vi "Autonomous Independent.vi"() -> ()   [LabVIEW 2019]
doc: "This VI is called when autonomous begins, and will automatically be terminated when autonomous ends. You can carry out timed or sensor driven robot movement independently without needing to return to the caller."
uses:
  <vilib>/Rock Robotics/WPI/Utilities/WPI_GetSetVariantRefNum.vi
  <vilib>/Rock Robotics/Network Tables/NT Write Numeric Array.vi
  <vilib>/Rock Robotics/Network Tables/NT Read String.vi
panel:
  out "Ultrasonic 2":dbl
  out "Ultrasonic":dbl
  out "Degrees 2":dbl(knob) scale=0.0..360.0
  out "Degrees":dbl(knob) scale=0.0..360.0
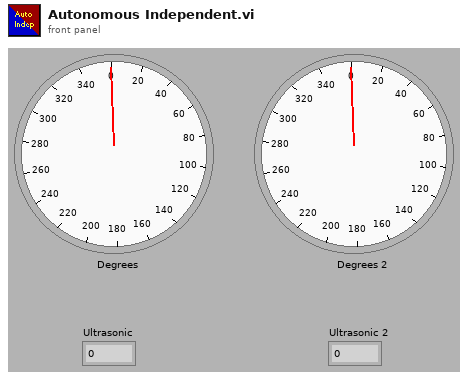
[diagram p1: front panel]
types:
  T1 = typedef "WPI_JoystickDevRef.ctl" = cluster{"Device":T2}
  T2 = typedef "WPI_JoystickDeviceEnum.ctl" = enum16{"USB 0", "USB 1", "USB 2", "USB 3", "USB 4", "USB 5"}
  T3 = typedef "WPI_RobotDriveDevRef.ctl" = cluster{"DevStatus":errorcluster, "Motors[]":T4[], "Square Inputs":bool, "Max Output":dbl}
  T4 = typedef "WPI_MotorControlDeviceRef.ctl" = cluster{"DeviceStatus":errorcluster, "Type":T5, "PWM":cluster{"PWM Channel":T6, "DeadBand":T7}, "CAN":cluster{"Device Number":u8, "SetOutput VI Ref":variant, "GetOutput VI Ref":variant, "Enable VI Ref":variant, "Disable VI Ref":variant, "Data":variant}, "Invert":bool, "DIO PWM":cluster{"PWM \"Enable\" Channel":T6, "DIOChannel":T8, "PWM Rate":dbl}}
  T5 = typedef "WPI_MotorControlType.ctl" = enum16{"PWM", "CAN", "DIO PWM"}
  T6 = typedef "FPGA_DIOPWMChannel.ctl" = enum8{"PWM 0", "PWM 1", "PWM 2", "PWM 3", "PWM 4", "PWM 5", "PWM 6", "PWM 7", "PWM 8", "PWM 9", "PWM MXP 0", "PWM MXP 1", "PWM MXP 2", "PWM MXP 3", "PWM MXP 4", "PWM MXP 5", "PWM MXP 6", "PWM MXP 7", "PWM MXP 8", "PWM MXP 9", "Invalid"}
  T7 = typedef "WPI_PWMDeadband.ctl" = cluster{"Name":string, "maxPositivePwm":i32, "minPositivePwm":i32, "centerPwm":i32, "maxNegativePwm":i32, "minNegativePwm":i32, "angularRange":u16}
  T8 = typedef "FPGA_DIOChannel.ctl" = enum8{"DIO 0", "DIO 1", "DIO 2", "DIO 3", "DIO 4", "DIO 5", "DIO 6", "DIO 7", "DIO 8", "DIO 9", "DIO MXP 0", "DIO MXP 1", "DIO MXP 2", "DIO MXP 3", "DIO MXP 4", "DIO MXP 5", "DIO MXP 6", "DIO MXP 7", "DIO MXP 8", "DIO MXP 9", "DIO MXP 10", "DIO MXP 11", "DIO MXP 12", "DIO MXP 13", "DIO MXP 14", "DIO MXP 15", "SPI Port CS1", "SPI Port CS2", "SPI Port CS3", "SPI Port MISO", "SPI Port MOSI", "Invalid"}
  T9 = typedef "WPI_GyroDevRef.ctl" = cluster{"DevStatus":errorcluster, "Analog Channel":T10, "Gain (VoltsPerDegree/Second)":dbl, "Gyro Type":enum16{"Analog", "XRS450"}, "Handle":i32, "SPI Bus":T11, "Device Found":bool, "Sample Rate":dbl, "Calibrate On Open":bool, "Offset":dbl}
  T10 = typedef "FPGA_AIChannel.ctl" = enum8{"AI 0", "AI 1", "AI 2", "AI 3", "AI MXP 0", "AI MXP 1", "AI MXP 2", "AI MXP 3", "Invalid"}
  T11 = typedef "spi_bus.ctl" = enum16{"SPI On-Board, CS0", "SPI On-Board, CS1", "SPI On-Board, CS2", "SPI On-Board, CS3", "SPI MXP", "Invalid"}
  T12 = typedef "WPI_AnalogChannelDevRef.ctl" = cluster{"DevStatus":errorcluster, "Analog Channel":T10}
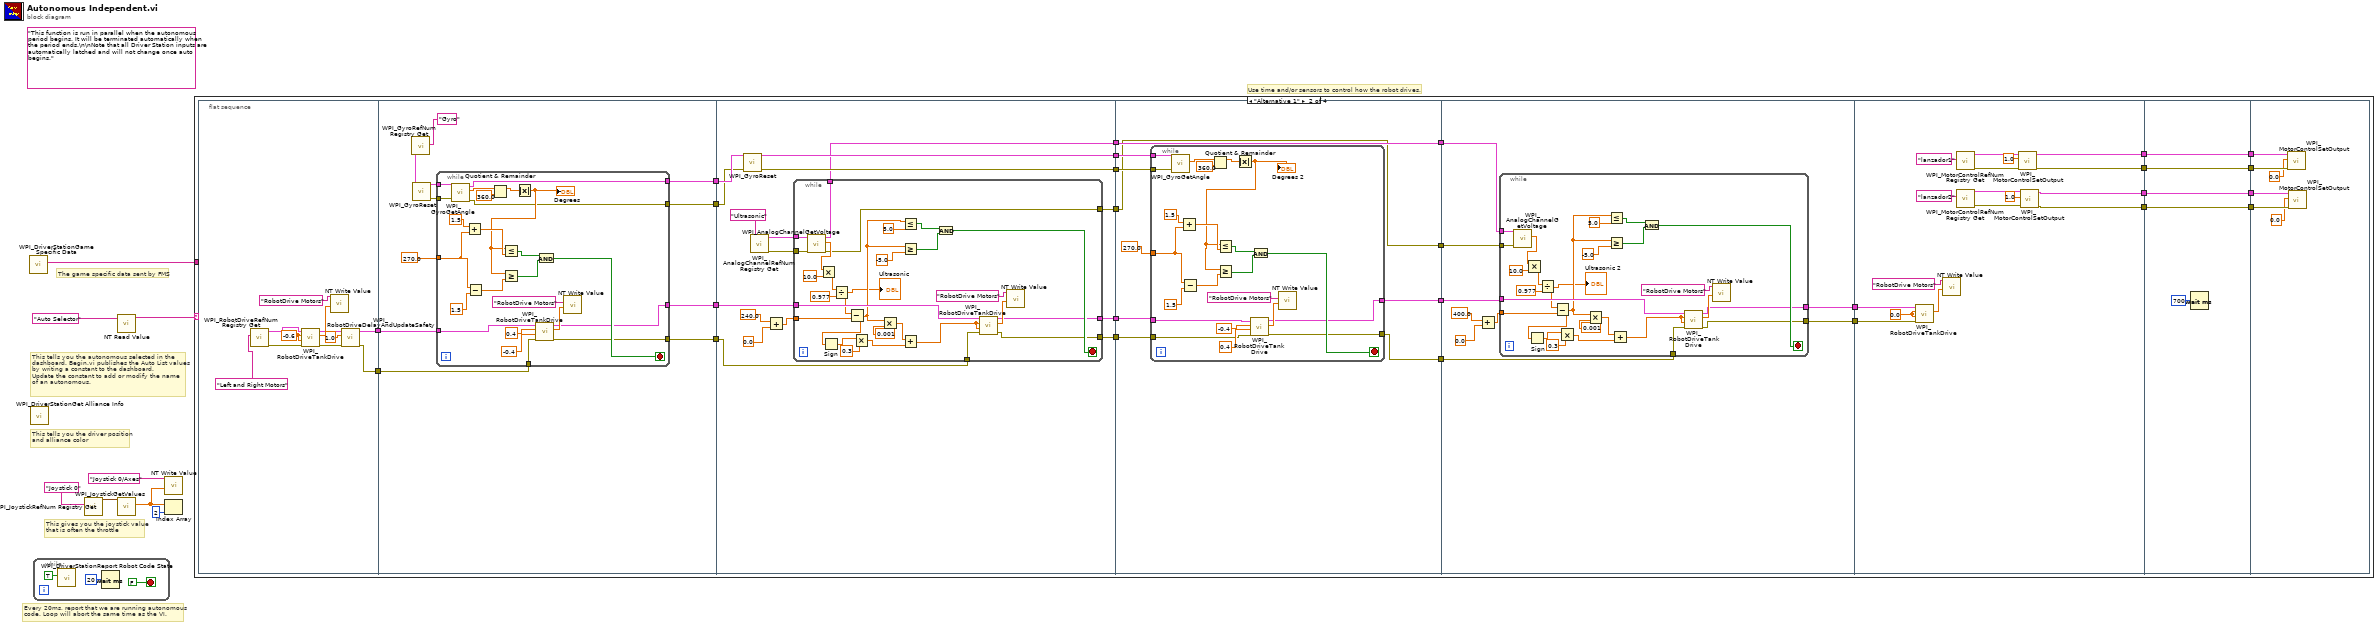
[diagram p0: block diagram]
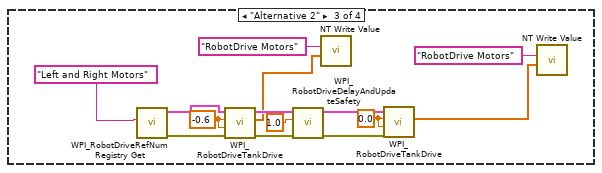
[diagram p3: hidden frame]
diagram:
  (unwired) "This function is run in parallel when the autonomous period begins. It will be terminated automatically when the period ends.\n\nNote that all Driver Station inputs are automatically latched and will not change once auto begins."
  # "The game specific data sent by FMS"
  # "This tells you the autonomous selected in the \ndashboard. Begin.vi publishes the Auto List values\nby writing a constant to the dashboard.\nUpdate the constant to add or modify the name\nof an autonomous."
  # "Every 20ms, report that we are running autonomous\ncode. Loop will abort the same time as the VI."
  # "This gives you the joystick value\nthat is often the throttle"
  # "Use time and/or sensors to control how the robot drives."
  # "This tells you the driver position\nand alliance color"
  n1 = call <vilib>:"WPI_DriverStationGame Specific Data.vi"() -> ("Game Specific Data"=w1:string)  [unwired: 11 in]
  n2 = call <vilib>:"WPI_DriverStationGet Alliance Info.vi"() -> ()  [unwired: 12 out]
  n3 = while {
    stop <- FALSE stop-if-true
    n4 = call <vilib>:"WPI_DriverStationReport Robot Code State.vi"("Autonomous"=TRUE) -> ()  [unwired: 10 in, 1 out]
    n5 = Wait (ms)(milliseconds to wait=u32 20) -> ()  [unwired: 1 out]
  }
  n6 = call <vilib>:"WPI_JoystickRefNum Registry Get.vi"("refnum name"="Joystick 0") -> ("JoystickDevRef"=w7:T1)  [unwired: 1 in, 9 out]
  n7 = call <vilib>:"WPI_JoystickGetValues.vi"("JoystickDevRef"=w7) -> ("Axes"=w3:dbl[])  [unwired: 6 in, 4 out]
  n8 = call-poly <vilib>:"NT Read Value.vi"("Name"="Auto Selector") -> ("String"=w4:string)  [unwired: 9 in, 1 out]
  n9 = call-poly <vilib>:"NT Write Value.vi"("Numeric Array"=w3, "Name"="Joystick 0/Axes") -> ()  [unwired: 9 in, 1 out]
  n10 = Index Array(array=w3, index=2) -> ()  [unwired: 1 out]
  n11 = case shown="\"Alternative 1\"" w4 {
    tunnel: w1 -> [_ _ _ _]
    frame Default {
      # "You can put your main auto here, or you can right-click on the case and make any\nother frame be the default case."
      # "This is the frame that will execute if no selection is made, or if it is not recognized"
    }
    frame "Alternative 1" {
      n12 = flat-sequence {
        tunnel: [w41] -> w13
        tunnel: [w42] -> w12
        tunnel: [w54] -> w37
        tunnel: [w53] -> w36
        tunnel: [w52] -> w35
        tunnel: [w51] -> w34
        tunnel: w13 -> [w50]
        tunnel: w12 -> [w49]
        tunnel: w37 -> [w94]
        tunnel: w36 -> [w93]
        tunnel: w35 -> [w92]
        tunnel: w34 -> [w91]
        tunnel: [w90] -> w33
        tunnel: [w89] -> w32
        tunnel: [w88] -> w31
        tunnel: [w87] -> w30
        tunnel: [w86] -> w26
        tunnel: [w85] -> w24
        tunnel: w33 -> [w137]
        tunnel: w32 -> [w136]
        tunnel: w31 -> [w134]
        tunnel: w30 -> [w133]
        tunnel: [w132] -> w29
        tunnel: [w131] -> w28
        tunnel: [w130] -> w27
        tunnel: w26 -> [w130]
        tunnel: [w129] -> w25
        tunnel: w24 -> [w129]
        tunnel: w29 -> [w168]
        tunnel: w28 -> [w164]
        tunnel: w27 -> [w163]
        tunnel: w25 -> [w162]
        tunnel: [w161] -> w23
        tunnel: [w160] -> w22
        tunnel: w23 -> [w201]
        tunnel: w22 -> [w200]
        tunnel: [w198] -> w20
        tunnel: [w197] -> w18
        tunnel: [w196] -> w16
        tunnel: [w195] -> w14
        tunnel: [w215] -> w21
        tunnel: w20 -> [w215]
        tunnel: [w214] -> w19
        tunnel: w18 -> [w214]
        tunnel: [w213] -> w17
        tunnel: w16 -> [w213]
        tunnel: [w212] -> w15
        tunnel: w14 -> [w212]
        tunnel: w21 -> [w222]
        tunnel: w19 -> [w221]
        tunnel: w17 -> [w220]
        tunnel: w15 -> [w219]
        frame #0 {
          w48 = -0.6 ("Left axis value")
          n13 = call <vilib>:"WPI_RobotDriveRefNum Registry Get.vi"("refnum name"="Left and Right Motors") -> ("error out"=w46:errorcluster, "RobotDriveDevRef"=w47:T3)  [unwired: 9 in]
          n14 = call <vilib>:"WPI_RobotDriveTankDrive.vi"("error in (no error)"=w46, "Right axis value"=w48, "Left axis value"=w48, "RobotDriveDevRef"=w47) -> ("error out"=w44:errorcluster, "Motor Values"=w38:dbl[], "RobotDriveDevRef"=w45:T3)  [unwired: 5 in]
          n15 = call-poly <vilib>:"NT Write Value.vi"("Numeric Array"=w38, "Name"="RobotDrive Motors") -> ()  [unwired: 9 in, 1 out]
          n16 = call <vilib>:"WPI_RobotDriveDelayAndUpdateSafety.vi"("error in (no error)"=w44, "Delay (s)"=1.0, "RobotDriveDevRef"=w45) -> ("error out"=w41:errorcluster, "RobotDriveDevRef 2"=w42:T3)  [unwired: 7 in]
        }
        frame #1 {
          n17 = call <vilib>:"WPI_GyroRefNum Registry Get.vi"("refnum name"="Gyro") -> ("error out"=w58:errorcluster, "GyroDevRef"=w59:T9)  [unwired: 9 in]
          n18 = call <vilib>:"WPI_GyroReset.vi"("error in"=w58, "GyroDevRef"=w59) -> ("error out"=w56:errorcluster, "GyroDevRef"=w57:T9)  [unwired: 8 in]
          n19 = while {
            tunnel: w57 -> [w84]
            tunnel: w56 -> [w83]
            tunnel: 270.0 ("y") -> [w75]
            tunnel: [w66] -> w54
            tunnel: [w65] -> w53
            tunnel: [w64] -> w52
            tunnel: [w63] -> w51
            tunnel: w50 -> [w62]
            tunnel: w49 -> [w61]
            stop <- w78 stop-if-true
            n20 = call <vilib>:"WPI_GyroGetAngle.vi"("error in"=w83, "GyroDevRef"=w84) -> ("error out"=w63:errorcluster, "Angle"=w70:dbl, "GyroDevRef"=w64:T9)  [unwired: 5 in, 2 out]
            n21 = Add(x=1.5 ("y"), y=w75) -> (x+y=w71:dbl)
            n22 = Subtract(x=w75, y=1.5 ("x")) -> (x-y=w72:dbl)
            n23 = Quotient & Remainder(x=w70, y=360.0) -> (x-y*floor(x/y)=w68:dbl)  [unwired: 1 out]
            n24 = Absolute Value(x=w68) -> (abs(x)=w67:dbl)
            "Degrees" <- w67
            n25 = Less Or Equal?(x=w67, y=w71) -> (x <= y?=w73:bool)
            n26 = Greater Or Equal?(x=w67, y=w72) -> (x >= y?=w74:bool)
            n27 = call <vilib>:"WPI_RobotDriveTankDrive.vi"("error in (no error)"=w62, "Right axis value"=-0.4 ("X axis value"), "Left axis value"=0.4 ("X axis value"), "RobotDriveDevRef"=w61) -> ("error out"=w65:errorcluster, "Motor Values"=w82:dbl[], "RobotDriveDevRef"=w66:T3)  [unwired: 5 in]
            n28 = And(x=w73, y=w74) -> (x .and. y?=w78:bool)
            n29 = call-poly <vilib>:"NT Write Value.vi"("Numeric Array"=w82, "Name"="RobotDrive Motors") -> ()  [unwired: 9 in, 1 out]
          }
        }
        frame #2 {
          n30 = call <vilib>:"WPI_GyroReset.vi"("error in"=w91, "GyroDevRef"=w92) -> ("error out"=w87:errorcluster, "GyroDevRef"=w88:T9)  [unwired: 8 in]
          n31 = call <vilib>:"WPI_AnalogChannelRefNum Registry Get.vi"("refnum name"="Ultrasonic") -> ("error out"=w99:errorcluster, "AIDeviceRef"=w98:T12)  [unwired: 9 in]
          n32 = Add(x=240.0 ("y"), y=0.0) -> (x+y=w95:dbl)
          n33 = while {
            tunnel: w99 -> [w124]
            tunnel: w98 -> [w123]
            tunnel: w95 -> [w122]
            tunnel: w94 -> [w117]
            tunnel: w93 -> [w113]
            tunnel: [w105] -> w90
            tunnel: [w104] -> w89
            tunnel: [w102] -> w86
            tunnel: [w101] -> w85
            stop <- w109 stop-if-true
            n34 = call <vilib>:"WPI_AnalogChannelGetVoltage.vi"("error in (no error)"=w124, "AIDeviceRef"=w123) -> ("error out"=w101:errorcluster, "Voltage"=w127:dbl, "AIDeviceRef"=w102:T12)  [unwired: 7 in]
            n35 = Multiply(x=w127, y=10.0) -> (x*y=w128:dbl)
            n36 = Divide(x=w128, y=0.977) -> (x/y=w103:dbl)
            "Ultrasonic" <- w103
            n37 = Subtract(x=w103, y=w122) -> (x-y=w106:dbl)
            n38 = Sign(1:w106) -> (0:w116:dbl)
            n39 = Multiply(x=w116, y=0.3) -> (x*y=w114:dbl)
            n40 = Multiply(x=w106, y=0.001) -> (x*y=w120:dbl)
            n41 = Less Or Equal?(x=w106, y=5.0 ("x")) -> (x <= y?=w111:bool)
            n42 = Greater Or Equal?(x=w106, y=-5.0 ("x")) -> (x >= y?=w110:bool)
            n43 = Add(x=w120, y=w114) -> (x+y=w112:dbl)
            n44 = And(x=w111, y=w110) -> (x .and. y?=w109:bool)
            n45 = call <vilib>:"WPI_RobotDriveTankDrive.vi"("error in (no error)"=w113, "Right axis value"=w112, "Left axis value"=w112, "RobotDriveDevRef"=w117) -> ("error out"=w105:errorcluster, "Motor Values"=w119:dbl[], "RobotDriveDevRef"=w104:T3)  [unwired: 5 in]
            n46 = call-poly <vilib>:"NT Write Value.vi"("Numeric Array"=w119, "Name"="RobotDrive Motors") -> ()  [unwired: 9 in, 1 out]
          }
        }
        frame #3 {
          n47 = while {
            tunnel: w136 -> [w155]
            tunnel: w137 -> [w154]
            tunnel: 270.0 ("y") -> [w150]
            tunnel: [w142] -> w132
            tunnel: [w141] -> w131
            tunnel: w134 -> [w138]
            tunnel: w133 -> [w139]
            stop <- w153 stop-if-true
            n48 = call <vilib>:"WPI_GyroGetAngle.vi"("error in"=w139, "GyroDevRef"=w138) -> ("Angle"=w145:dbl)  [unwired: 5 in, 4 out]
            n49 = Add(x=1.5 ("y"), y=w150) -> (x+y=w146:dbl)
            n50 = Subtract(x=w150, y=1.5 ("x")) -> (x-y=w147:dbl)
            n51 = Quotient & Remainder(x=w145, y=360.0) -> (x-y*floor(x/y)=w143:dbl)  [unwired: 1 out]
            n52 = Absolute Value(x=w143) -> (abs(x)=w140:dbl)
            "Degrees 2" <- w140
            n53 = Less Or Equal?(x=w140, y=w146) -> (x <= y?=w148:bool)
            n54 = Greater Or Equal?(x=w140, y=w147) -> (x >= y?=w149:bool)
            n55 = call <vilib>:"WPI_RobotDriveTankDrive.vi"("error in (no error)"=w154, "Right axis value"=0.4 ("X axis value"), "Left axis value"=-0.4 ("X axis value"), "RobotDriveDevRef"=w155) -> ("error out"=w141:errorcluster, "Motor Values"=w159:dbl[], "RobotDriveDevRef"=w142:T3)  [unwired: 5 in]
            n56 = And(x=w148, y=w149) -> (x .and. y?=w153:bool)
            n57 = call-poly <vilib>:"NT Write Value.vi"("Numeric Array"=w159, "Name"="RobotDrive Motors") -> ()  [unwired: 9 in, 1 out]
          }
        }
        frame #4 {
          n58 = Add(x=400.0 ("y"), y=0.0) -> (x+y=w165:dbl)
          n59 = while {
            tunnel: w162 -> [w190]
            tunnel: w163 -> [w189]
            tunnel: w165 -> [w188]
            tunnel: w168 -> [w183]
            tunnel: w164 -> [w179]
            tunnel: [w170] -> w161
            tunnel: [w169] -> w160
            stop <- w175 stop-if-true
            n60 = call <vilib>:"WPI_AnalogChannelGetVoltage.vi"("error in (no error)"=w190, "AIDeviceRef"=w189) -> ("Voltage"=w193:dbl)  [unwired: 7 in, 2 out]
            n61 = Multiply(x=w193, y=10.0) -> (x*y=w194:dbl)
            n62 = Divide(x=w194, y=0.977) -> (x/y=w171:dbl)
            "Ultrasonic 2" <- w171
            n63 = Subtract(x=w171, y=w188) -> (x-y=w172:dbl)
            n64 = Sign(1:w172) -> (0:w182:dbl)
            n65 = Multiply(x=w182, y=0.3) -> (x*y=w180:dbl)
            n66 = Multiply(x=w172, y=0.001) -> (x*y=w186:dbl)
            n67 = Less Or Equal?(x=w172, y=5.0 ("x")) -> (x <= y?=w177:bool)
            n68 = Greater Or Equal?(x=w172, y=-5.0 ("x")) -> (x >= y?=w176:bool)
            n69 = Add(x=w186, y=w180) -> (x+y=w178:dbl)
            n70 = And(x=w177, y=w176) -> (x .and. y?=w175:bool)
            n71 = call <vilib>:"WPI_RobotDriveTankDrive.vi"("error in (no error)"=w179, "Right axis value"=w178, "Left axis value"=w178, "RobotDriveDevRef"=w183) -> ("error out"=w169:errorcluster, "Motor Values"=w185:dbl[], "RobotDriveDevRef"=w170:T3)  [unwired: 5 in]
            n72 = call-poly <vilib>:"NT Write Value.vi"("Numeric Array"=w185, "Name"="RobotDrive Motors") -> ()  [unwired: 9 in, 1 out]
          }
        }
        frame #5 {
          w199 = 0.0 ("Left axis value")
          n73 = call <vilib>:"WPI_RobotDriveTankDrive.vi"("error in (no error)"=w200, "Right axis value"=w199, "Left axis value"=w199, "RobotDriveDevRef"=w201) -> ("Motor Values"=w203:dbl[])  [unwired: 5 in, 2 out]
          n74 = call-poly <vilib>:"NT Write Value.vi"("Numeric Array"=w203, "Name"="RobotDrive Motors") -> ()  [unwired: 9 in, 1 out]
          n75 = call <vilib>:"WPI_MotorControlRefNum Registry Get.vi"("refnum name"="lanzador1") -> ("error out"=w210:errorcluster, "MotorControlDevRef"=w211:T4)  [unwired: 9 in]
          n76 = call <vilib>:"WPI_MotorControlRefNum Registry Get.vi"("refnum name"="lanzador2") -> ("error out"=w206:errorcluster, "MotorControlDevRef"=w207:T4)  [unwired: 9 in]
          n77 = call <vilib>:"WPI_MotorControlSetOutput.vi"("error in (no error)"=w210, "Output"=1.0, "MotorControlDevRef"=w211) -> ("error out"=w195:errorcluster, "MotorControlDevRef"=w198:T4)  [unwired: 6 in, 1 out]
          n78 = call <vilib>:"WPI_MotorControlSetOutput.vi"("error in (no error)"=w206, "Output"=1.0, "MotorControlDevRef"=w207) -> ("error out"=w196:errorcluster, "MotorControlDevRef"=w197:T4)  [unwired: 6 in, 1 out]
        }
        frame #6 {
          n79 = Wait (ms)(milliseconds to wait=u32 700) -> ()  [unwired: 1 out]
        }
        frame #7 {
          n80 = call <vilib>:"WPI_MotorControlSetOutput.vi"("error in (no error)"=w219, "Output"=0.0, "MotorControlDevRef"=w222) -> ()  [unwired: 6 in, 3 out]
          n81 = call <vilib>:"WPI_MotorControlSetOutput.vi"("error in (no error)"=w220, "Output"=0.0, "MotorControlDevRef"=w221) -> ()  [unwired: 6 in, 3 out]
        }
      }
    }
    frame "Alternative 2" {
      w227 = 0.0 ("Left axis value")
      w236 = -0.6 ("Left axis value")
      n82 = call <vilib>:"WPI_RobotDriveRefNum Registry Get.vi"("refnum name"="Left and Right Motors") -> ("error out"=w234:errorcluster, "RobotDriveDevRef"=w235:T3)  [unwired: 9 in]
      n83 = call <vilib>:"WPI_RobotDriveTankDrive.vi"("error in (no error)"=w234, "Right axis value"=w236, "Left axis value"=w236, "RobotDriveDevRef"=w235) -> ("error out"=w232:errorcluster, "Motor Values"=w224:dbl[], "RobotDriveDevRef"=w233:T3)  [unwired: 5 in]
      n84 = call <vilib>:"WPI_RobotDriveDelayAndUpdateSafety.vi"("error in (no error)"=w232, "Delay (s)"=1.0, "RobotDriveDevRef"=w233) -> ("error out"=w228:errorcluster, "RobotDriveDevRef 2"=w229:T3)  [unwired: 7 in]
      n85 = call-poly <vilib>:"NT Write Value.vi"("Numeric Array"=w224, "Name"="RobotDrive Motors") -> ()  [unwired: 9 in, 1 out]
      n86 = call <vilib>:"WPI_RobotDriveTankDrive.vi"("error in (no error)"=w228, "Right axis value"=w227, "Left axis value"=w227, "RobotDriveDevRef"=w229) -> ("Motor Values"=w223:dbl[])  [unwired: 5 in, 2 out]
      n87 = call-poly <vilib>:"NT Write Value.vi"("Numeric Array"=w223, "Name"="RobotDrive Motors") -> ()  [unwired: 9 in, 1 out]
    }
    frame "Stellar" {
    }
  }
